vi "TimeNumberMatchMarcoGonzalez.vi"() -> ()   [LabVIEW 2012]
panel:
  out "Time":dbl
  out "Number Found":dbl
  in  "Numeric":dbl
  in  "0 to:":dbl
  out "# of Guesses":dbl
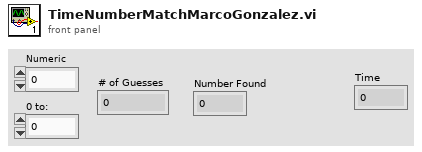
[diagram p1: front panel]
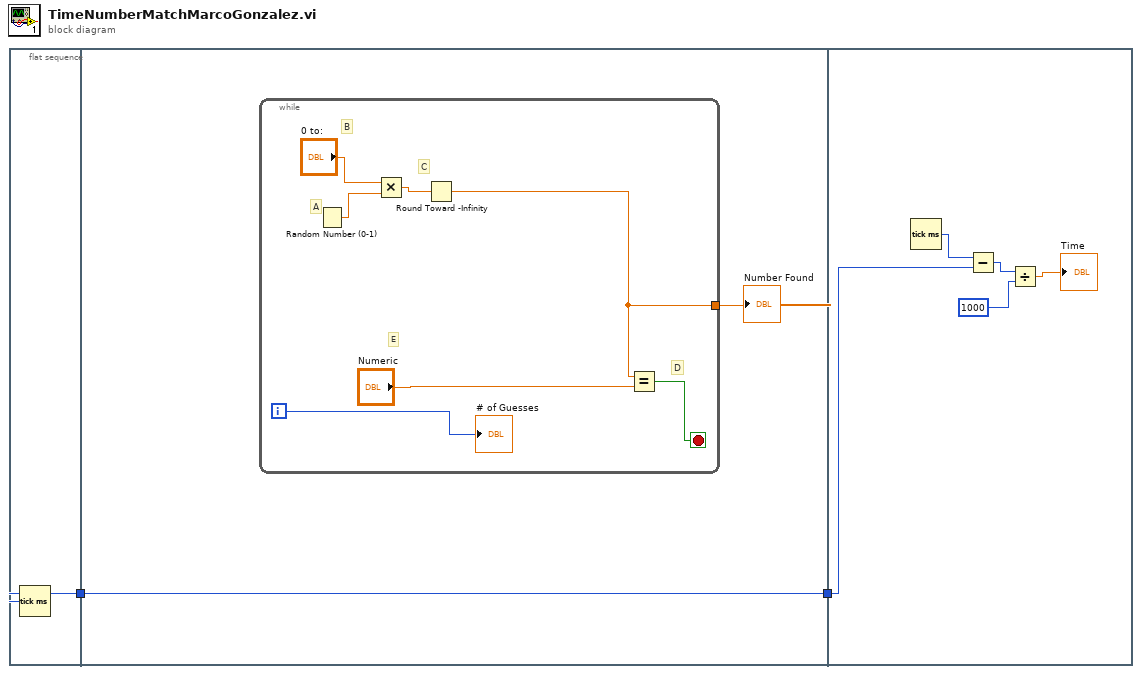
[diagram p0: block diagram]
diagram:
  n1 = flat-sequence {
    tunnel: [w3] -> w1
    tunnel: [w4] -> w2
    tunnel: w1 -> [w4]
    tunnel: w2 -> [w15]
    frame #0 {
      n2 = Tick Count (ms)() -> (millisecond timer value=w3:u32)
    }
    frame #1 {
      n3 = while {
        tunnel: [w8] -> w5
        i -> [w6]
        stop <- w7 stop-if-true
        # "E"
        # "D"
        # "C"
        # "B"
        # "A"
        n4 = Random Number (0-1)() -> (number: 0 to 1=w10:dbl)
        n5 = Multiply(x="0 to:", y=w10) -> (x*y=w9:dbl)
        n6 = Round Toward -Infinity(1:w9) -> (0:w8:dbl)
        n7 = Equal?(x=w8, y="Numeric") -> (x = y?=w7:bool)
        "# of Guesses" <- w6
      }
      "Number Found" <- w5
    }
    frame #2 {
      n8 = Tick Count (ms)() -> (millisecond timer value=w17:u32)
      n9 = Subtract(x=w17, y=w15) -> (x-y=w14:u32)
      n10 = Divide(x=w14, y=1000) -> (x/y=→"Time":dbl)
    }
  }
